vi "view variant in tree helper.vi"(4 "is array element?":bool, 6 "index string":string, 8 "error in (no error)":errorcluster, 9 "Item Indent":i32, 10 "Variant":variant, 11 "Items":T1(array[cluster])) -> (0 "error out":errorcluster, 3 "Items out":T1(array[cluster]))   [LabVIEW 2017, in "DSF Configuration Utility.lvlib"]
uses:
  DSF Configuration.llb/DSF Configuration Utility.lvlib
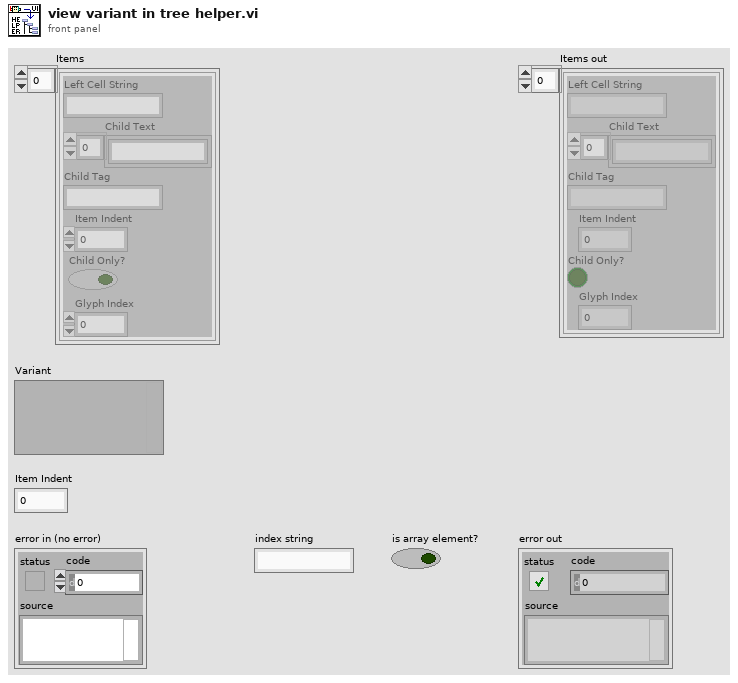
[diagram p1: front panel]
types:
  T1 = cluster{"Left Cell String":string, "Child Text":string[], "Child Tag":string, "Item Indent":i32, "Child Only?":bool, "Glyph Index":i32}[]
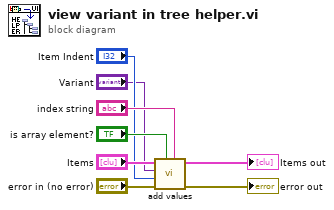
[diagram p0: block diagram]
diagram:
  n1 = call "add values.vi"("index string"="index string", "is array element?"="is array element?", "error in (no error)"="error in (no error)", "Item Indent"="Item Indent", "Variant"="Variant", "Items in"="Items") -> ("error out"=→"error out":errorcluster, "Items out"=→"Items out":T1)  [unwired: 4 in]
